vi "Goal_Tensions_FGV.vi"(10 "Write Goal Tension":dbl[](array[numeric]), 11 "Operation":enum16{"Write", "Read"}(ring)) -> (3 "Read Goal Tension":dbl[](array[numeric]))   [LabVIEW 2024]
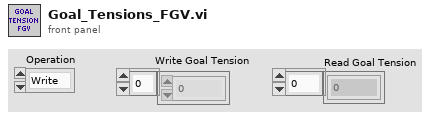
[diagram p1: front panel]
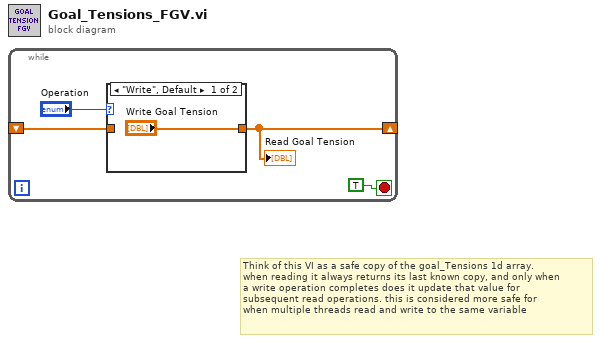
[diagram p0: block diagram]
diagram:
  # "Think of this VI as a safe copy of the goal_Tensions 1d array.\nwhen reading it always returns its last known copy, and only when\na write operation completes does it update that value for \nsubsequent read operations. this is considered more safe for \nwhen multiple threads read and write to the same variable"
  n1 = while {
    shift-right: [w2] -> _
    shift-left: _ -> [w3]
    stop <- TRUE stop-if-true
    n2 = case shown="\"Write\", Default" "Operation" {
      tunnel: w3 -> [_ w6]
      tunnel: ["Write Goal Tension" w6] -> w2
      frame "Write", Default {
      }
      frame "Read" {
      }
    }
    "Read Goal Tension" <- w2
  }
